vi "Error Messages.vi"(8 "error in (no error)":errorcluster) -> (2 "Error Substring":string, 3 "message":string=" INSTRUCTIONS:\r\rNormal Use:  When using subVIs that incorporate the error in/error out (or error I/O) structure, place this handler where you want to inform the user of an error, typically at the end of the I/O data path, as the last action of the program.  If the error in error? is ERROR, the handler creates a message describing the error and its source.  If the type of dialog = 1 (default), the message is displayed to the user, who can only acknowedge it.  If the type = 2, the user can acknowledge the message or abort execution; aborting a program with active I/O is not recommended.  If the type = 0, no message is displayed; this is used to process the error programmatically, and the error out cluster elements are wired to individual terminals for that reason.  \r\rOther Use:\n\r\nlocal testing.  To test the error code of a subVI or function that does not have the error I/O structure, you can wire its error code and a source string to the local error code and error source inputs.  If error in error? indicates no error and error code is not equal to 0, the local code and source are substituted for the error in values, and error? is set TRUE (ERROR).")   [LabVIEW 2012, in "OpenCLV x64.lvlib"]
doc: "Error handling VI specifcally for OpenCLV. When available, OpenCL errors have been used. To make these errors compliant with Labview, -5000 has been added to the error. For example, CL_DEVICE_NOT_FOUND is normaly -1, but in OpenCLV it is -5001."
uses:
  OpenCLV x64.lvlib
  <vilib>/Utility/error.llb/DialogType.ctl
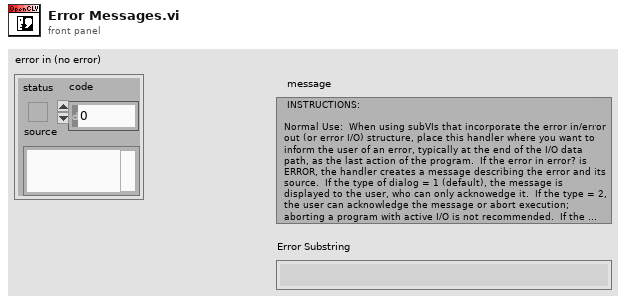
[diagram p1: front panel]
types:
  T1 = typedef "DialogType.ctl" = u16
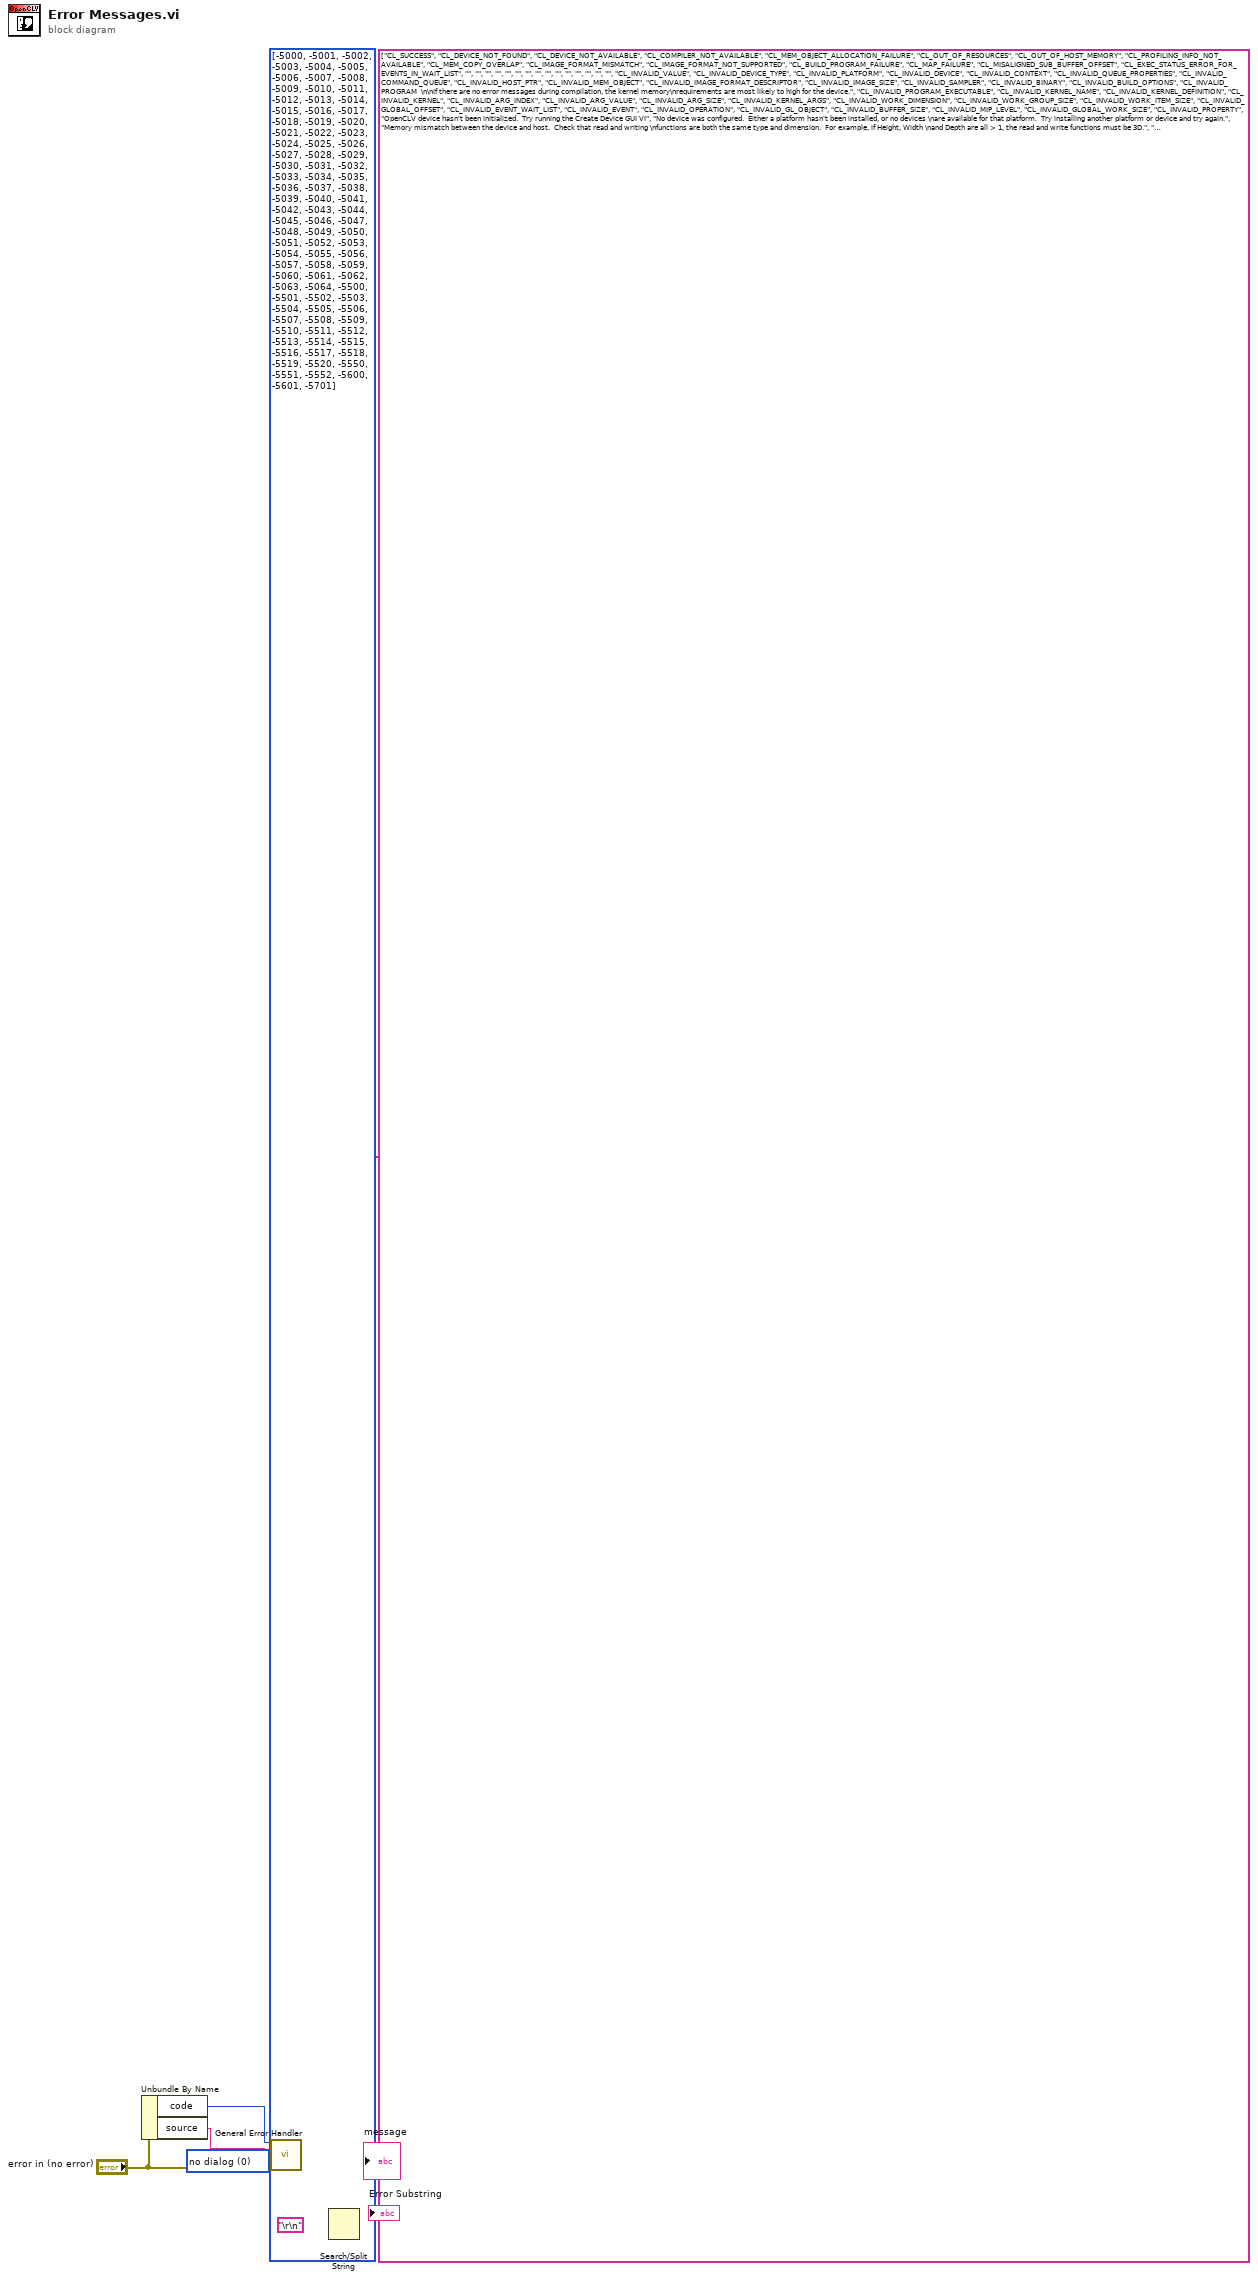
[diagram p0: block diagram]
diagram:
  w6 = T1 0 items=["no dialog", "OK message", "continue or stop message", "OK message + warnings", "continue/stop + warnings"] ("type of dialog (OK msg:1)")
  n1 = Unbundle By Name("error in (no error)") -> ("code"=w7:i32, "source"=w5:string)
  n2 = call <vilib>:"General Error Handler.vi"("[error code] (0)"=w7, "[user-defined codes]"=i32[] [-5000, -5001, -5002, -5003, -5004, -5005, -5006, -5007, -5008, -5009, -5010, -5011, -5012, -5013, -5014, -5015, -5016, -5017, -5018, -5019, -5020, -5021, -5022, -5023, -5024, -5025, -5026, -5027, -5028, -5029, -5030, -5031, -5032, -5033, -5034, -5035, -5036, -5037, -5038, -5039, -5040, -5041, -5042, -5043, -5044, -5045, -5046, -5047, -5048, -5049, -5050, -5051, -5052, -5053, -5054, -5055, -5056, -5057, -5058, -5059, -5060, -5061, -5062, -5063, -5064, -5500, -5501, -5502, -5503, -5504, -5505, -5506, -5507, -5508, -5509, -5510, -5511, -5512, -5513, -5514, -5515, -5516, -5517, -5518, -5519, -5520, -5550, -5551, -5552, -5600, -5601, -5701] ("Array"), "[user-defined descriptions]"=string[] ["CL_SUCCESS", "CL_DEVICE_NOT_FOUND", "CL_DEVICE_NOT_AVAILABLE", "CL_COMPILER_NOT_AVAILABLE", "CL_MEM_OBJECT_ALLOCATION_FAILURE", "CL_OUT_OF_RESOURCES", "CL_OUT_OF_HOST_MEMORY", "CL_PROFILING_INFO_NOT_AVAILABLE", "CL_MEM_COPY_OVERLAP", "CL_IMAGE_FORMAT_MISMATCH", "CL_IMAGE_FORMAT_NOT_SUPPORTED", "CL_BUILD_PROGRAM_FAILURE", "CL_MAP_FAILURE", "CL_MISALIGNED_SUB_BUFFER_OFFSET", "CL_EXEC_STATUS_ERROR_FOR_EVENTS_IN_WAIT_LIST", "", "", "", "", "", "", "", "", "", "", "", "", "", "", "", "CL_INVALID_VALUE", "CL_INVALID_DEVICE_TYPE", "CL_INVALID_PLATFORM", "CL_INVALID_DEVICE", "CL_INVALID_CONTEXT", "CL_INVALID_QUEUE_PROPERTIES", "CL_INVALID_COMMAND_QUEUE", "CL_INVALID_HOST_PTR", "CL_INVALID_MEM_OBJECT", "CL_INVALID_IMAGE_FORMAT_DESCRIPTOR", "CL_INVALID_IMAGE_SIZE", "CL_INVALID_SAMPLER", "CL_INVALID_BINARY", "CL_INVALID_BUILD_OPTIONS", "CL_INVALID_PROGRAM  \n\nIf there are no error messages during compilation, the kernel memory\nrequirements are most likely to high for the device.", "CL_INVALID_PROGRAM_EXECUTABLE", "CL_INVALID_KERNEL_NAME", "CL_INVALID_KERNEL_DEFINITION", "CL_INVALID_KERNEL", "CL_INVALID_ARG_INDEX", "CL_INVALID_ARG_VALUE", "CL_INVALID_ARG_SIZE", "CL_INVALID_KERNEL_ARGS", "CL_INVALID_WORK_DIMENSION", "CL_INVALID_WORK_GROUP_SIZE", "CL_INVALID_WORK_ITEM_SIZE", "CL_INVALID_GLOBAL_OFFSET", "CL_INVALID_EVENT_WAIT_LIST", "CL_INVALID_EVENT", "CL_INVALID_OPERATION", "CL_INVALID_GL_OBJECT", "CL_INVALID_BUFFER_SIZE", "CL_INVALID_MIP_LEVEL", "CL_INVALID_GLOBAL_WORK_SIZE", "CL_INVALID_PROPERTY", "OpenCLV device hasn't been initialized.  Try running the Create Device GUI VI", "No device was configured.  Either a platform hasn't been installed, or no devices \nare available for that platform.  Try installing another platform or device and try again.", "Memory mismatch between the device and host.  Check that read and writing \nfunctions are both the same type and dimension.  For example, if Height, Width \nand Depth are all > 1, the read and write functions must be 3D.", "An array dimension is 0.  Only values of 1 and high are acceptable.  Try using \nthe Array Dimensions.ctl to prevent accidental input values.", "OPENCLV_CANT_INIT_FFT_FRAMEWORK", "OPENCLV_CANT_DESTROY_FFT_FRAMEWORK", "OPENCLV_FFT_FAILED", "OPENCLV_FFT_BUFFER_FAILED", "OPENCLV_FFT_GET_BUFF_SIZE_FAILED", "OPENCLV_FFT_GET_LAYOUT_FAILED", "OPENCLV_FFT_PLAN_DESTROY_FAILED", "OPENCLV_FFT_DEFAULT_PLAN_FAILED", "OPENCLV_FFT_SET_RESULT_FAILED", "OPENCLV_FFT_SET_LAYOUT_FAILED", "OPENCLV_FFT_SET_BATCHSIZE_FAILED", "OPENCLV_FFT_SET_STRIDES_IN_FAILED", "OPENCLV_FFT_SET_STRIDES_OUT_FAILED", "OPENCLV_FFT_SET_PLAN_DIST_FAILED", "OPENCLV_FFT_BAKE_PLAN_FAILED", "OPENCLV_FFT_SET_PRECISION_FAILED", "OPENCLV_FFT_INVALID_PLAN", "Memory is either mapped and being used with un-mapped memory functions or vice versa.", "Memory is not mapped.  Try mapping the memory or using unmapped memroy functions.", "Memory types do not match.  For example, memory was allocated as 32f, but is \nbeing read as 64f memory.  Please check the data types and try again.", "QR Matrix decompostion requires a square matrix.", "The kernel dimensions all need to be non-zero and odd.", "The kernel encountered a runtime error.  Most likely this is caused by read-write \nerrors or accessing memory outside of that designated."], "[error source] (\" \")"=w5, "type of dialog (OK msg:1)"=w6, "error in (no error)"="error in (no error)") -> ("message"=w3:string)  [unwired: 5 in, 4 out]
  "message" <- w3
  n3 = Search/Split String(string=w3, search string/char (-)="\r\n") -> (substring before match=→"Error Substring":string)  [unwired: 1 in, 2 out]
